vi "Write Dataset with Attributes (Variant).vi"(4 "Data":variant, 5 "Attribute Names":string[](array[string]), 6 "operation (open or create)":T1=enum."open or create", 7 "Attribute Values":variant[](array[variant]), 8 "error in (no error)":errorcluster, 9 "Unlimited  dataset (F)":bool, 10 "Dataset Path":string, 11 "HDF5 Ref":T2) -> (0 "error out":errorcluster, 3 "HDF5 Ref out":T2)   [LabVIEW 2017]
doc: "Writes data into a dataset along with some attributes."
uses:
  <vilib>/UPVI/lvhdf5/library.llb/HDF5 Ref.ctl
  <vilib>/UPVI/lvhdf5/dataset.llb/LVH5D Operation.ctl
  <vilib>/UPVI/lvhdf5/attribute.llb/LVH5A Operation.ctl
panel:
  # "LVHDF5 Toolkit\nCopyright (c) 2005-2013 by Jason D. Sommerville\nCopyright (c) 2014 by UPVI, LLC.\n\nThis use and distribution of this file is governed by the terms found in \nLICENSE.txt distributed with this toolkit and installed at\n <user.lib>\\_lvhdf5\\LICENSE.txt"
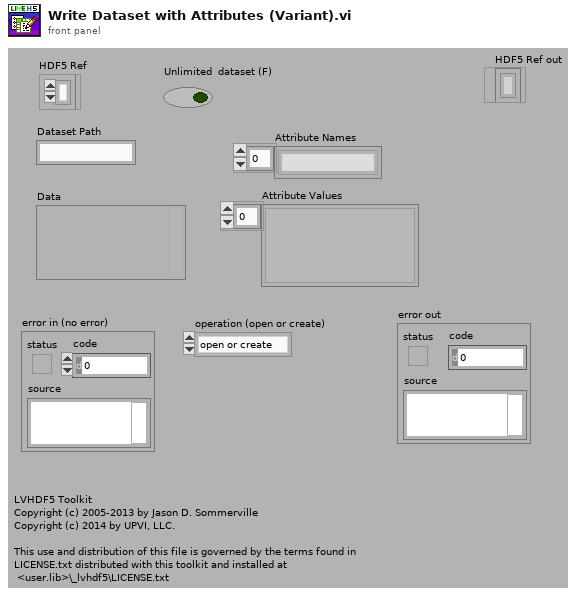
[diagram p1: front panel]
types:
  T1 = typedef "LVH5D Operation.ctl" = enum16{"open", "replace", "create", "open or create", "create or replace", "create or replace with confirmation"}
  T2 = typedef "HDF5 Ref.ctl" = refnum<k1>
  T3 = typedef "LVH5A Operation.ctl" = enum16{"open", "replace", "create", "open or create", "create or replace", "create or replace with confirmation"}
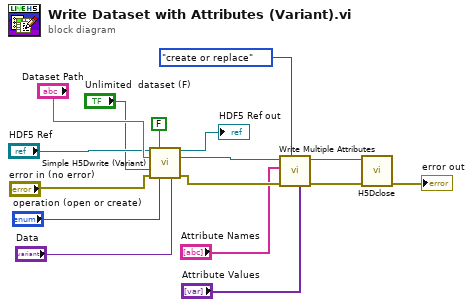
[diagram p0: block diagram]
diagram:
  n1 = call <vilib>:"Simple H5Dwrite (Variant).vi"("HDF5 Location Ref"="HDF5 Ref", "Close Dataset (T)"=FALSE, "Dataset Path"="Dataset Path", "Unlimited  dataset (F)"="Unlimited  dataset (F)", "error in (no error)"="error in (no error)", "operation (open or create)"="operation (open or create)", "Data"="Data") -> ("HDF5 Location Ref out"=→"HDF5 Ref out":T2, "HDF5 Dataset Ref out"=w12:T2, "error out"=w13:errorcluster)  [unwired: 6 in]
  n2 = call <vilib>:"Write Multiple Attributes.vi"("Values"="Attribute Values", "operation (open or create)"=LVH5A_Operation."create or replace", "error in (no error)"=w13, "Names"="Attribute Names", "HDF5 Ref"=w12) -> ("error out"=w14:errorcluster, "HDF5 Ref out"=w16:T2)  [unwired: 3 in]
  n3 = call <vilib>:"H5Dclose.vi"("error in (no error)"=w14, "HDF5 Dataset Ref"=w16) -> ("error out"=→"error out":errorcluster)  [unwired: 7 in]
